vi "NotifyObserver.vi"(8 "error in (no error)":errorcluster, 10 "Variant":variant, 11 "Observable in":refnum<class "Observable.lvclass">) -> (0 "error out":errorcluster, 3 "Observable out":refnum<class "Observable.lvclass">)   [LabVIEW 2013, in "Observable.lvclass"]
uses:
  Observable.lvclass
  Observable.lvclass/Observable.ctl
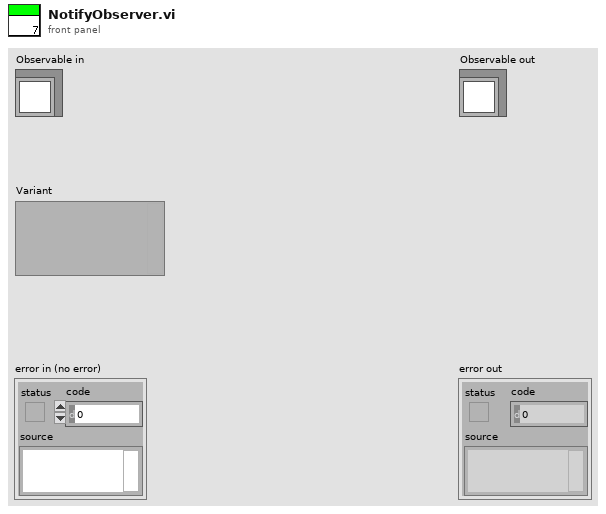
[diagram p1: front panel]
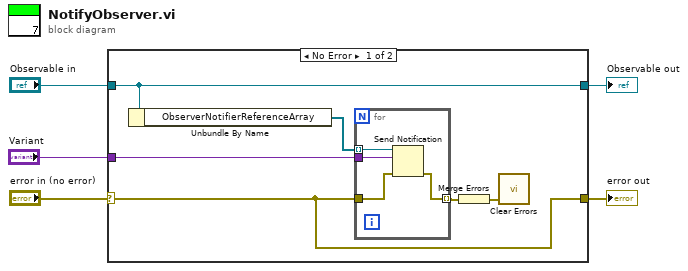
[diagram p0: block diagram]
diagram:
  n1 = case shown="No Error" "error in (no error)" {
    selector: "error in (no error)" -> [w6 w16]
    tunnel: [w6 w16] -> w1
    tunnel: [w10 w17] -> w3
    tunnel: "Observable in" -> [w10 w17]
    tunnel: "Variant" -> [w11 _]
    frame No Error {
      n2 = Unbundle By Name(w10) -> ("ObserverNotifierReferenceArray"=w9:refnum<notifier>[])
      n3 = for {
        tunnel: w9 -> [w15] mode=indexing
        tunnel: w6 -> [w13]
        tunnel: [w12] -> w8 mode=indexing
        tunnel: w11 -> [w14]
        n4 = Send Notification(notification=w14, notifier=w15, error in (no error)=w13) -> (error out=w12:errorcluster)  [unwired: 1 out]
      }
      n5 = Merge Errors(w8) -> (w7:errorcluster)
      n6 = call <vilib>:"Clear Errors.vi"("error in (no error)"=w7) -> ()  [unwired: 6 in, 1 out]
    }
    frame Error {
    }
  }
  "error out" <- w1
  "Observable out" <- w3
